vi "WaitForReceipt.vi"(8 "error in (no error)":errorcluster, 9 "timeout in ms (10000)":i32=10000, 11 "STOMP in":refnum<class "STOMP.lvclass">) -> (0 "error out":errorcluster, 2 "receipt":T1, 3 "STOMP out":refnum<class "STOMP.lvclass">)   [LabVIEW 2017, in "LabVIEW STOMP.lvlib" / "STOMP.lvclass"]
uses:
  STOMP.lvclass
  Typedefs/Type_ServerFrame.ctl
  Typedefs/Type_ServerFrameType.ctl
  STOMP.lvclass/STOMP.ctl
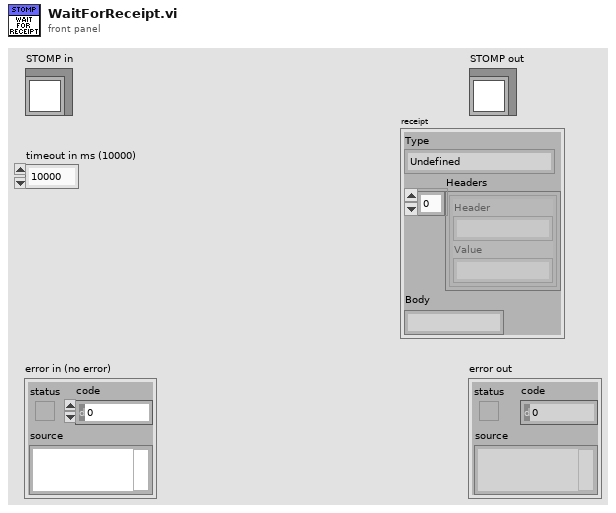
[diagram p1: front panel]
types:
  T1 = typedef "LabVIEW STOMP.lvlib/STOMP.lvclass/Type_ServerFrame.ctl" = cluster{"Type":T2, "Headers":cluster{"Header":string, "Value":string}[], "Body":string}
  T2 = typedef "LabVIEW STOMP.lvlib/STOMP.lvclass/Type_ServerFrameType.ctl" = enum16{"Undefined", "MESSAGE", "CONNECTED", "RECEIPT", "ERROR"}
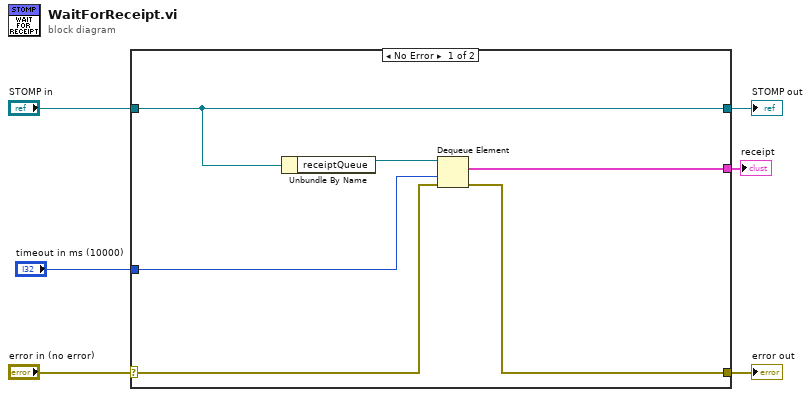
[diagram p0: block diagram]
diagram:
  n1 = case shown="No Error" "error in (no error)" {
    selector: "error in (no error)" -> [w10 w14]
    tunnel: [w7 w14] -> w5
    tunnel: [w12 w13] -> w3
    tunnel: "STOMP in" -> [w12 w13]
    tunnel: "timeout in ms (10000)" -> [w9 _]
    tunnel: [w8 _] -> w1
    frame No Error {
      n2 = Unbundle By Name(w12) -> ("receiptQueue"=w11:refnum<queue>)
      n3 = Dequeue Element(queue=w11, timeout in ms (-1)=w9, error in (no error)=w10) -> (element=w8:T1, error out=w7:errorcluster)  [unwired: 2 out]
    }
    frame Error {
    }
  }
  "error out" <- w5
  "STOMP out" <- w3
  "receipt" <- w1
